vi "Handle Request Error.vi"(8 "Request Error":errorcluster, 11 "WriteRequest in":refnum<class "WriteRequest.lvclass">) -> ()   [LabVIEW 2019, in "MessagingInterfaces.lvlib" / "WriteRequest.lvclass"]
uses:
  <vilib>/gpm_packages/@cs/Network-interface/Source/MessagingInterfaces/WriteRequest/WriteRequest.lvclass
  <vilib>/gpm_packages/@cs/Network-interface/Source/MessagingInterfaces/WriteRequest/WriteRequest.lvclass/WriteRequest.ctl
  <vilib>/gpm_packages/@cs/Network-interface/Source/MessagingInterfaces/IWriteExecutionCallback/IWriteExecutionCallback.lvclass
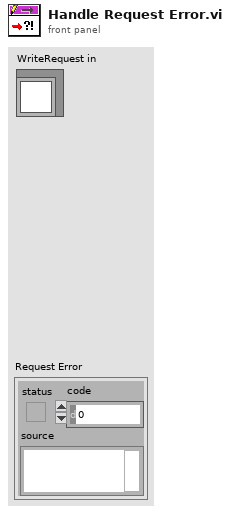
[diagram p1: front panel]
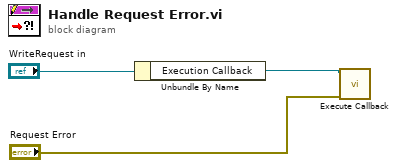
[diagram p0: block diagram]
diagram:
  n1 = Unbundle By Name("WriteRequest in") -> ("Execution Callback"=w2:refnum<class "IWriteExecutionCallback.lvclass">)
  n2 = call-dynamic "Execute Callback.vi"("Write Status"="Request Error", "IWriteExecutionPolicy in"=w2) -> ()  [unwired: 10 in]
